vi "Eagle_RT LED Ring Intensity.vi"() -> ()   [LabVIEW 2015]
uses:
  <vilib>/FPGAPlugInAG/cRIO-9030/niLvFpga_Open_cRIO-9030.vi
  <vilib>/rvi/interface/common/dynamic/niFpgaDynamicAddResources.vi
  <vilib>/FPGAPlugInAG/Dynamic/niLvFpga_Run_Dynamic.vi
  Eagle_RT Globals.vi
  <vilib>/Utility/error.llb/Error Cluster From Error Code.vi
  <vilib>/rvi/errors/niLvFpgaAdjustHostInterfaceError.vi
  <vilib>/rvi/interface/nirviOpenFPGA/nirviOpenFPGA.xnode
  FPGA Bitfiles/BELKINEAGLEGUI_FPGATarget_EagleFPGAIntensi_ZYNfgiSn2nQ.lvbitx
  <vilib>/rvi/interface/nirviMethod/nirviMethod.xnode
  <vilib>/rvi/interface/nirviReadWriteControl/nirviReadWriteControl.xnode
  NiFpgaLv.dll
  <vilib>/rvi/interface/Simulation/niFpgaSimulationCallBeginRW.vi
panel:
  in  "Mode":enum16{"OFF", "ON"}(ring)
  in  "LR Intensity":fxp<+,16,3>
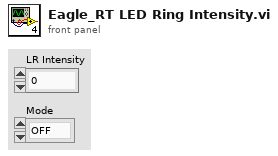
[diagram p1: front panel]
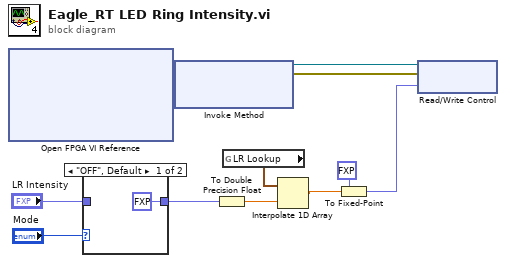
[diagram p0: block diagram]
diagram:
  n1 = xnode "Open FPGA VI Reference"() -> ("FPGA VI Reference Out"=w12:refnum<k20>, "error out"=w9:errorcluster)  [unwired: 2 in]
  n2 = case shown="\"OFF\", Default" "Mode" {
    tunnel: [fxp<+,16,3> 0.0 ("RB Intensity") w14] -> w1
    tunnel: "LR Intensity" -> [_ w14]
    frame "OFF", Default {
    }
    frame "ON" {
    }
  }
  n3 = xnode "Invoke Method"("FPGA VI Reference In"=w12, "error in"=w9) -> ("FPGA VI Reference Out"=w11:refnum<k20>, "error out"=w10:errorcluster)  [unwired: 1 in]
  n4 = To Double Precision Float(number=w1) -> (double precision float=w7:dbl)
  n5 = global read "Eagle_RT Globals.vi" "LR Lookup"() -> (w8:cluster{"x":dbl, "y":dbl}[])
  n6 = Interpolate 1D Array(1:w7, 2:w8) -> (0:w6:dbl)
  n7 = To Fixed-Point(fixed-point type=fxp<+,16,3> 0.0, number=w6) -> (fixed-point=w4:fxp<+,16,3>)
  n8 = xnode "Read/Write Control"("FPGA VI Reference In"=w11, "error in"=w10, "LR Intensity"=w4) -> ()  [unwired: 2 out]
